vi "CreateCluster.vi"(8 "error in (no error)":errorcluster, 10 "ChildTypes":refnum<class "LVType.lvclass">[](array[class]), 11 "ID":string) -> (0 "error out":errorcluster, 3 "LVClusterType out":refnum<class "LVClusterType.lvclass">)   [LabVIEW 2020, in "LVDataTypes.lvlib" / "LVClusterType.lvclass"]
uses:
  <vilib>/AppBuilder/Engine/WebServiceDescription/LVDataTypes/LVClusterType/LVClusterType.lvclass
  e:/builds/penguin/labview/branches/2020/dev/dist/vi.lib/AppBuilder/Engine/WebServiceDescription/LVDataTypes/LVType/LVType.lvclass
  <vilib>/AppBuilder/Engine/WebServiceDescription/LVDataTypes/LVType/LVType.lvclass
  <vilib>/AppBuilder/Engine/WebServiceDescription/LVDataTypes/TypeCode.ctl
  <vilib>/AppBuilder/Engine/WebServiceDescription/LVDataTypes/LVClusterType/LVClusterType.lvclass/LVClusterType.ctl
  <vilib>/AppBuilder/Engine/WebServiceDescription/LVDataTypes/LVDataTypes.lvlib
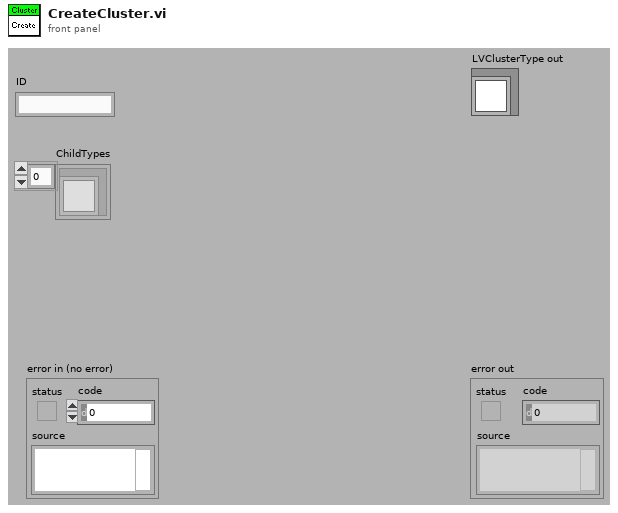
[diagram p1: front panel]
types:
  T1 = typedef "LVDataTypes.lvlib/TypeCode.ctl" = enum16{"Undefined", "Byte", "Unsigned Byte", "Word", "Unsigned Word", "Long", "Unsigned Long", "Quad", "Unsigned Quad", "Single", "Double", "Extended", "Enum", "Boolean", "String", "Path", "Array", "Cluster", "AnalogWaveform", "DigitalWaveform", "Time Stamp", "Void", "Complex Single", "Complex Double", "Complex Extended"}
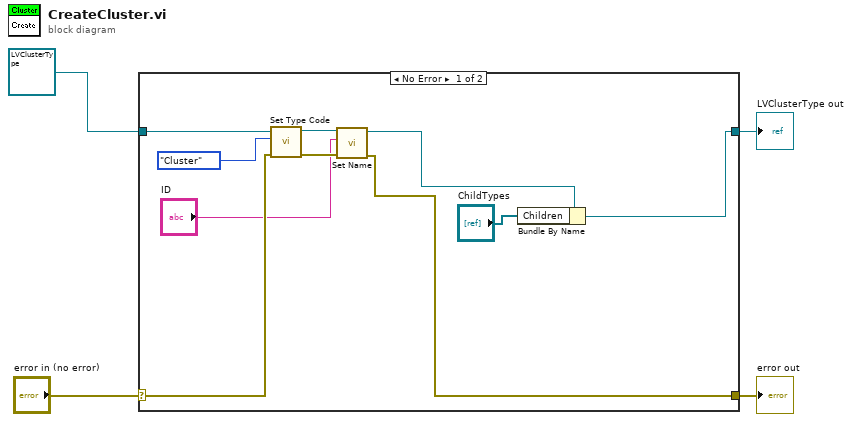
[diagram p0: block diagram]
diagram:
  n1 = case shown="No Error" "error in (no error)" {
    selector: "error in (no error)" -> [w10 w16]
    tunnel: [w6 w16] -> w3
    tunnel: [w13 w15] -> w1
    tunnel: refnum<class "LVClusterType.lvclass"> refnum ("LVClusterType in") -> [w12 w15]
    frame No Error {
      n2 = call <vilib>:"Set Type Code.vi"("error in (no error)"=w10, "Type"=TypeCode."Cluster", "LVType.lvclass in"=w12) -> ("error out"=w9:errorcluster, "LVType.lvclass out"=w8:refnum<class "LVClusterType.lvclass">)  [unwired: 7 out]
      n3 = call <vilib>:"Set Name.vi"("error in (no error)"=w9, "Name"="ID", "LVType.lvclass in"=w8) -> ("error out"=w6:errorcluster, "LVType.lvclass out"=w5:refnum<class "LVClusterType.lvclass">)  [unwired: 7 out]
      n4 = Bundle By Name(cluster=w5, "Children"="ChildTypes") -> (w13:refnum<class "LVClusterType.lvclass">)
    }
    frame Error {
    }
  }
  "error out" <- w3
  "LVClusterType out" <- w1
